vi "EvaluateConditions.vi"(7 "map":T1, 8 "error in":errorcluster, 9 "force burst":bool, 10 "device":string, 11 "burst mode trigger":variant) -> (0 "error out":errorcluster, 1 "reason":string, 2 "burst":bool, 3 "burst mode trigger":variant)   [LabVIEW 2017, in "BurstMode.lvlib"]
uses:
  <vilib>/addons/InsightCM/Devices/Shared/Cms/CmsBurstMode/BurstMode.lvlib
  <vilib>/addons/PointValueMap/controls/PointMap.ctl
  <vilib>/addons/InsightCM/Devices/Shared/Cms/CmsBurstMode/controls/device.ctl
  <vilib>/addons/InsightCM/MessageBus/Base/controls/KeyValuePair.ctl
  <vilib>/addons/InsightCM/Devices/Shared/Common/Trigger/controls/TriggerCondition.ctl
  <vilib>/addons/InsightCM/MessageBus/Base/controls/Condition.ctl
  <vilib>/addons/InsightCM/Devices/Shared/Common/DataEventCreator/controls/Reason.ctl
  <vilib>/addons/PointValueMap/subVIs/Point_Write_double.vi
  <vilib>/addons/InsightCM/Devices/Shared/Common/Trigger/Trigger.lvlib
  <vilib>/addons/InsightCM/Devices/Shared/Common/DataEventCreator/DataEventCreator.lvlib
  <vilib>/addons/PointValueMap/PointValueMap.lvlib
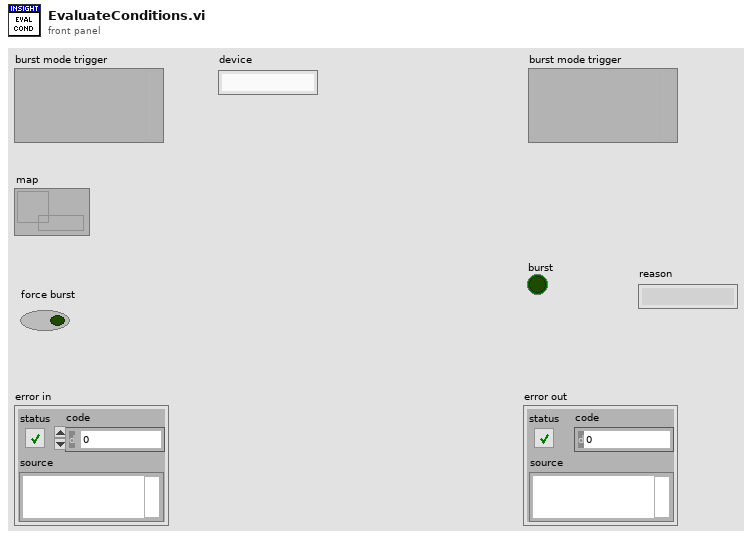
[diagram p1: front panel]
types:
  T1 = typedef "PointValueMap.lvlib/PointMap.ctl" = refnum<data-value>
  T2 = typedef "BurstMode.lvlib/device.ctl" = cluster{"Name":string, "Properties":T3[], "BurstExpression":string, "BurstConditions":T4[]}
  T3 = typedef "KeyValuePair.ctl" = cluster{"Key":string, "Value":string}
  T4 = typedef "Trigger.lvlib/TriggerCondition.ctl" = cluster{"Condition":T5, "LatchValue":string, "LatchTime":timestamp}
  T5 = typedef "Condition.ctl" = cluster{"Source":string, "Type":string, "Operator":string, "CompareTo":string, "DwellSeconds":dbl}
  T6 = typedef "DataEventCreator.lvlib/Reason.ctl" = enum16{"Periodic Event", "Delta EU Event", "Trend Event", "Alarm Event", "User Event", "Enter Operating State", "Exit Operating State", "Multiple Events", "Other"}
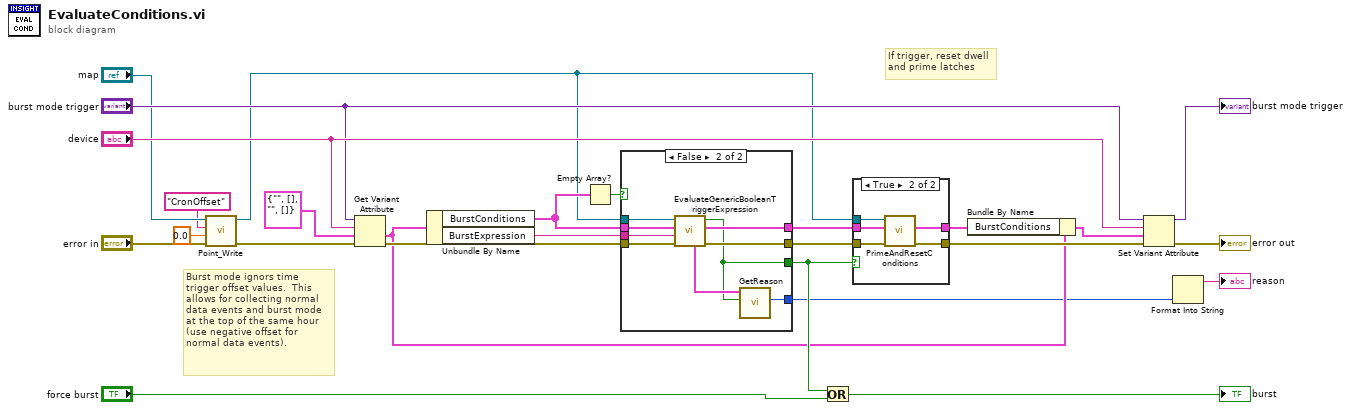
[diagram p0: block diagram]
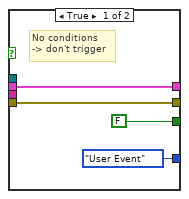
[diagram p3: hidden frame]
diagram:
  # "Burst mode ignors time\ntrigger offset values.  This\nallows for collecting normal\ndata events and burst mode\nat the top of the same hour \n(use negative offset for \nnormal data events)."
  # "If trigger, reset dwell\nand prime latches"
  n1 = call-poly <vilib>:"Point_Write.vi"("Error In"="error in", "Value"=0.0, "Tag"="CronOffset", "Map"="map") -> ("Error Out"=w1:errorcluster, "Map Out"=w5:T1)  [unwired: 6 in]
  n2 = Get Variant Attribute(Variant="burst mode trigger", name="device", default value (empty Variant)=T2 {"Name"="", "Properties"=[], "BurstExpression"="", "BurstConditions"=[]} ("Device Burst Mode"), error in=w1) -> (value=w12:T2, error out=w19:errorcluster)  [unwired: 2 out]
  n3 = Unbundle By Name(w12) -> ("BurstConditions"=w21:T4[], "BurstExpression"=w20:string)
  n4 = Empty Array?(array=w21) -> (empty?=w24:bool)
  n5 = case shown="False" w24 {
    tunnel: w20 -> [_ w39]
    tunnel: w19 -> [w29 w38]
    tunnel: [w29 w37] -> w25
    tunnel: [w28 w36] -> w23
    tunnel: w5 -> [_ w35]
    tunnel: [FALSE ("trigger") w32] -> w22
    tunnel: w21 -> [w28 w34]
    tunnel: [Reason."User Event" ("reason") w31] -> w7
    frame True {
      # "No conditions \n-> don't trigger"
    }
    frame False {
      n6 = call <vilib>:"EvaluateGenericBooleanTriggerExpression.vi"("error in (no error)"=w38, "expression"=w39, "all conditions"=w34, "map"=w35) -> ("error out"=w37:errorcluster, "all conditions out"=w36:T4[], "trigger"=w32:bool, "triggered conditions"=w33:T4[])  [unwired: 4 in]
      n7 = call <vilib>:"GetReason.vi"("condition met"=w32, "triggered conditions"=w33) -> ("reason"=w31:T6)  [unwired: 9 in]
    }
  }
  n8 = Or(x=w22, y="force burst") -> (x .or. y?=→"burst":bool)
  n9 = case shown="True" w22 {
    tunnel: w25 -> [w40 w44]
    tunnel: w23 -> [w41 w45]
    tunnel: [w40 w43] -> w15
    tunnel: w5 -> [_ w46]
    tunnel: [w41 w42] -> w11
    frame False {
    }
    frame True {
      n10 = call <vilib>:"PrimeAndResetConditions.vi"("error in (no error)"=w44, "conditions in"=w45, "SnapshotMap"=w46) -> ("error out"=w43:errorcluster, "conditions out"=w42:T4[])  [unwired: 7 in]
    }
  }
  n11 = Bundle By Name(cluster=w12, "BurstConditions"=w11) -> (w10:T2)
  n12 = Set Variant Attribute(Variant="burst mode trigger", name="device", value=w10, error in=w15) -> (Variant out=→"burst mode trigger":variant, error out=→"error out":errorcluster)  [unwired: 1 out]
  n13 = Format Into String(w7) -> (resulting string=→"reason":string)  [unwired: 3 in, 1 out]
